vi "Write Output directory.vi"(8 "error in (no error)":errorcluster, 10 "Output JSON File Path":path, 11 "FileConverterBase in":refnum<class "FileConverterBase.lvclass">) -> (0 "error out":errorcluster, 3 "FileConverterBase out":refnum<class "FileConverterBase.lvclass">)   [LabVIEW 2017, in "FileConverterBase.lvclass"]
uses:
  FileConverterBase.lvclass
  FileConverterBase.lvclass/FileConverterBase.ctl
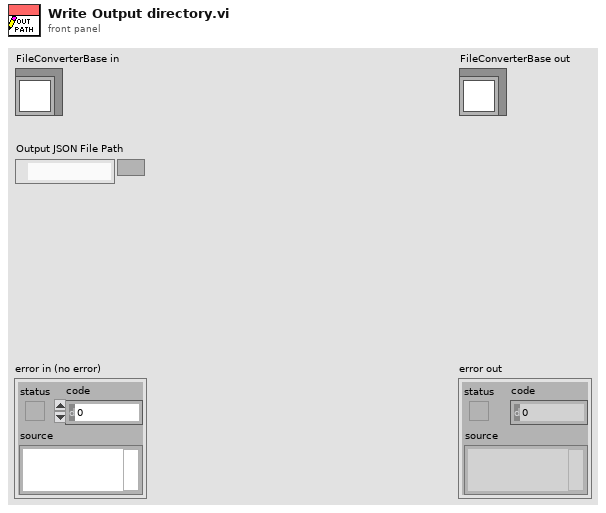
[diagram p1: front panel]
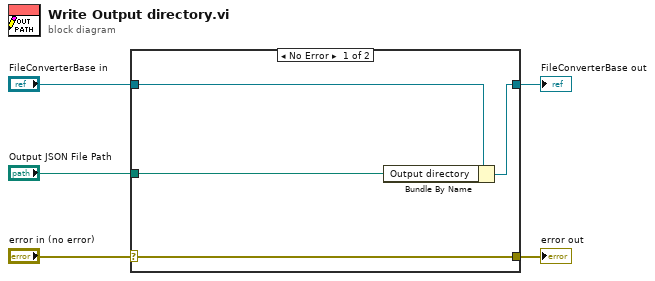
[diagram p0: block diagram]
diagram:
  n1 = case shown="No Error" "error in (no error)" {
    selector: "error in (no error)" -> [w9 w10]
    tunnel: [w9 w10] -> w4
    tunnel: [w7 w11] -> w2
    tunnel: "FileConverterBase in" -> [w8 w11]
    tunnel: "Output JSON File Path" -> [w6 _]
    frame No Error {
      n2 = Bundle By Name(cluster=w8, "Output directory"=w6) -> (w7:refnum<class "FileConverterBase.lvclass">)
    }
    frame Error {
    }
  }
  "error out" <- w4
  "FileConverterBase out" <- w2
